vi "ble_evt_connection_status.vi"(8 "error in (no error)":errorcluster, 11 "COM Bluegiga in":refnum<visa-resource-name>) -> (0 "error out":errorcluster, 2 "Connection Status":T1={"MAC Address"="", "cnx handle"=0, "cnx flags"=0, "Address Type"=125, "Connection Interval (ms)"=125, "Timeout(ms)"=125, "Latency"=0, "bonding handle"=0} {"Address Type" items=["Public", "Random"]}, 3 "COM Bluegiga out":refnum<visa-resource-name>)   [LabVIEW 2013]
uses:
  type_def/connection_status_bundle.ctl
  type_def/address_type.ctl
  type_def/message_class.ctl
  type_def/message_type.ctl
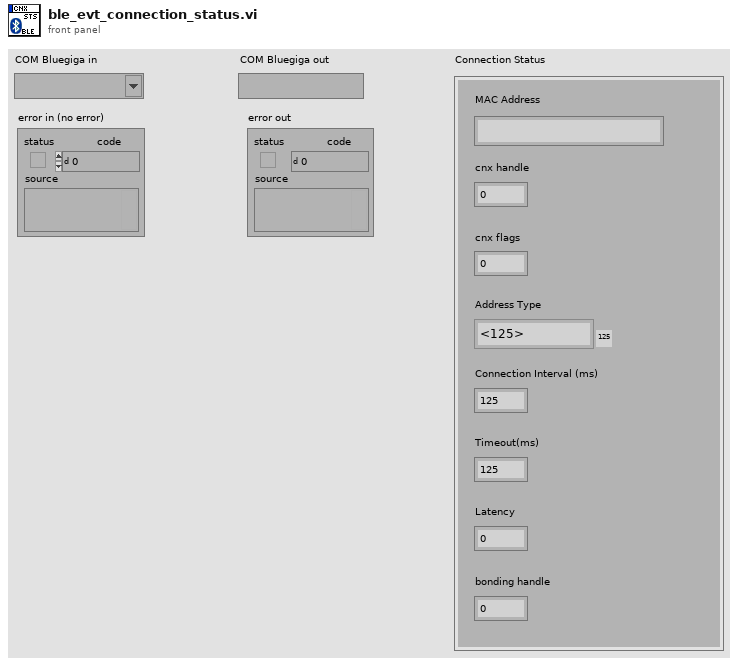
[diagram p1: front panel]
types:
  T1 = typedef "connection_status_bundle.ctl" = cluster{"MAC Address":string, "cnx handle":u8, "cnx flags":u8, "Address Type":T2, "Connection Interval (ms)":u16, "Timeout(ms)":u16, "Latency":u16, "bonding handle":u8}
  T2 = typedef "address_type.ctl" = u8
  T3 = typedef "message_type.ctl" = u8
  T4 = typedef "message_class.ctl" = u8
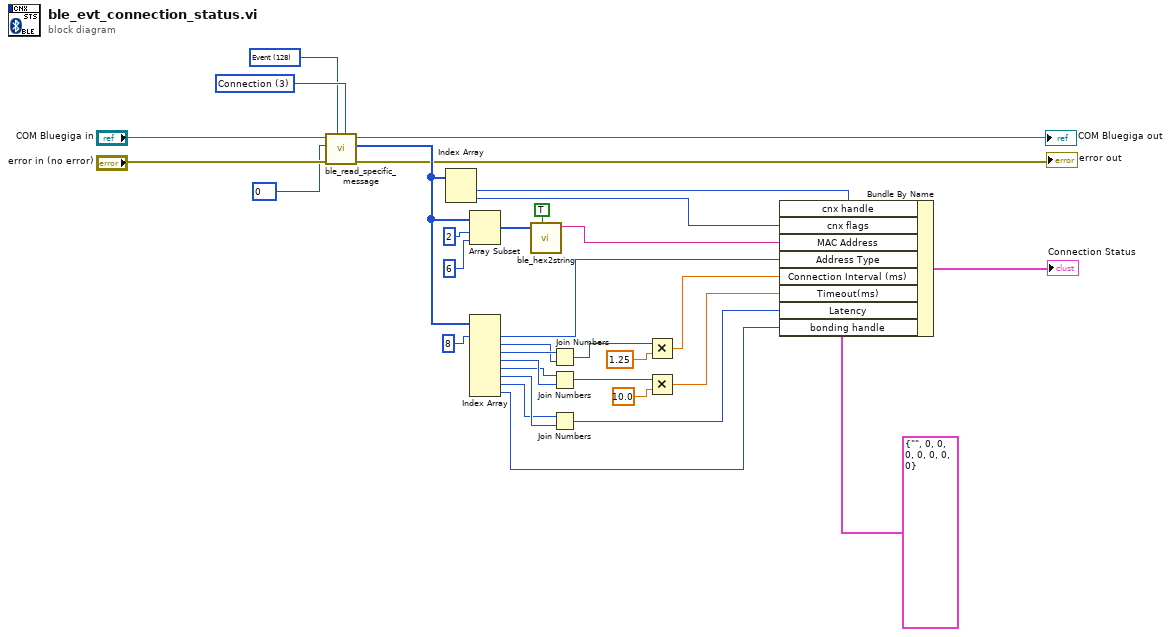
[diagram p0: block diagram]
diagram:
  w31 = T3 128 items=["Command / Response"=0, "Event"=128] ("Message Type (Response)")
  w32 = T4 3 items=["System", "Persistent Store", "Attribute database", "Connection", "Attribute client", "Security Manager", "Generic Access Profile", "Hardware"] ("Command Class (System)")
  n1 = call "ble_read_specific_message.vi"("Command Class (System)"=w32, "Message Type (Response)"=w31, "error in (no error)"="error in (no error)", "Message ID (0x00)"=u8 0, "COM Bluegiga in"="COM Bluegiga in") -> ("error out"=→"error out":errorcluster, "specific payload"=w26:u8[], "COM Bluegiga out"=→"COM Bluegiga out":refnum<visa-resource-name>)  [unwired: 2 in, 2 out]
  n2 = Index Array(array=w26) -> (element #1=w12:u8, element #2=w11:u8)  [unwired: 2 in]
  n3 = Array Subset(array=w26, index=2, length=6 ("index")) -> (w4:u8[])
  n4 = Index Array(array=w26, index #1=8 ("index")) -> (element #1=w10:u8, element #2=w22:u8, element #3=w23:u8, element #4=w20:u8, element #5=w19:u8, element #6=w18:u8, element #7=w17:u8, element #8=w6:u8)  [unwired: 7 in]
  n5 = call "ble_hex2string.vi"("colon?(false)"=TRUE, "Byte Array IN (index0 LS byte)"=w4) -> ("HEX string OUT"=w2:string)  [unwired: 9 in]
  n6 = Join Numbers(hi=w23, lo=w22) -> ((hi.lo)=w21:u16)
  n7 = Join Numbers(hi=w19, lo=w20) -> ((hi.lo)=w15:u16)
  n8 = Join Numbers(hi=w17, lo=w18) -> ((hi.lo)=w7:u16)
  n9 = Multiply(x=w21, y=1.25) -> (x*y=w9:dbl)
  n10 = Multiply(x=w15, y=10.0) -> (x*y=w8:dbl)
  n11 = Bundle By Name(cluster=T1 {"MAC Address"="", "cnx handle"=0, "cnx flags"=0, "Address Type"=0, "Connection Interval (ms)"=0, "Timeout(ms)"=0, "Latency"=0, "bonding handle"=0} ("Connection Status"), "cnx handle"=w12, "cnx flags"=w11, "MAC Address"=w2, "Address Type"=w10, "Connection Interval (ms)"=w9, "Timeout(ms)"=w8, "Latency"=w7, "bonding handle"=w6) -> (→"Connection Status":T1)
